vi "Day 7.2 - align crabs subs with increasing fuel cost - improved performance.vi"(11 "input":i32[](array[numeric])) -> (3 "output":i32)   [LabVIEW 2021]
panel:
  out "position":i32
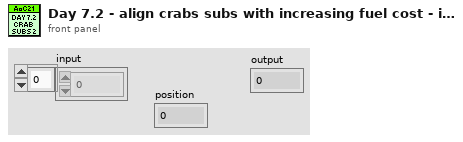
[diagram p1: front panel]
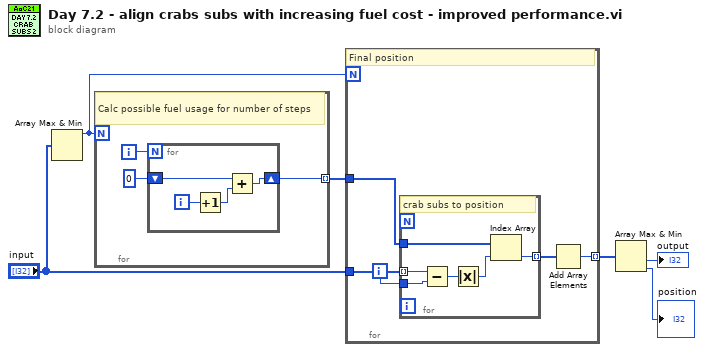
[diagram p0: block diagram]
diagram:
  n1 = Array Max & Min(array="input") -> (max value=w2:i32)  [unwired: 3 out]
  n2 = for {
    N: w2 -> [_]
    tunnel: [w7] -> w1 mode=indexing
    i -> [w8]
    # "Calc possible fuel usage for number of steps"
    n3 = for {
      N: w8 -> [_]
      shift-right: [w10] -> w7
      shift-left: 0 -> [w12]
      i -> [w13]
      n4 = Increment(x=w13) -> (x+1=w11:i32)
      n5 = Add(x=w12, y=w11) -> (x+y=w10:i32)
    }
  }
  n6 = for {
    N: w2 -> [_]
    tunnel: "input" -> [w18]
    tunnel: [w15] -> w5 mode=indexing
    tunnel: w1 -> [w14]
    i -> [w17]
    # "Final position"
    n7 = for {
      tunnel: w17 -> [w23]
      tunnel: w18 -> [w24] mode=indexing
      tunnel: [w20] -> w16 mode=indexing
      tunnel: w14 -> [w19]
      # "crab subs to position"
      n8 = Subtract(x=w24, y=w23) -> (x-y=w22:i32)
      n9 = Absolute Value(x=w22) -> (abs(x)=w21:i32)
      n10 = Index Array(array=w19, index=w21) -> (element=w20:i32)
    }
    n11 = Add Array Elements(numeric array=w16) -> (sum=w15:i32)
  }
  n12 = Array Max & Min(array=w5) -> (min value=→"output":i32, min index (indices)=→"position":i32)  [unwired: 2 out]
